vi "Connect LCR Relay.vi"(0 "reference in":refnum<class "NI-DAQmx.lvclass">, 2 "Relay Mode":enum16{"UV", "UW", "VW"}(ring), 5 "error in (no error)":errorcluster) -> (14 "reference out":refnum<class "NI-DAQmx.lvclass">, 19 "error out":errorcluster)   [LabVIEW 2018, in "NI-DAQmx.lvclass"]
uses:
  NI-DAQmx.lvclass
  <vilib>/DAQmx/write.llb/DAQmx Write (Digital 1D Bool NChan 1Samp 1Line).vi
  <vilib>/DAQmx/miscellaneous.llb/DAQmx Fill In Error Info.vi
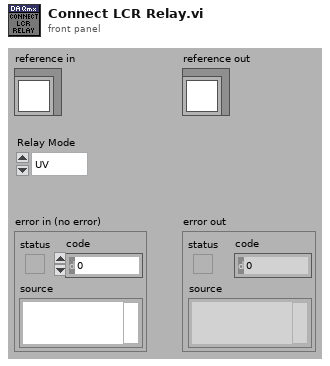
[diagram p1: front panel]
types:
  T1 = typedef "NI-DAQmx.lvclass/ObjectAttributes.ctl" = cluster{"AI Task":refnum<k21>, "DO Task":refnum<k21>, "AO Task":refnum<k21>, "Latest Values":dbl[], "Signal List":T2[], "PWM Duty Cycle (%)":dbl, "PWM Amplitude (V)":dbl, "PWM Frequency (Hz)":dbl, "DO States":bool[]}
  T2 = typedef "IO Signal List.ctl" = enum16{"Timestamp", "PSU_FB_U_VDC", "PSU_FB_I_AMP", "PSU_FB_W_WATT", "PSU_CMD_U_VDC", "PSU_CMD_I_AMP", "PSU_CMD_OUTPUT", "U_U_VDC", "V_U_VDC", "W_U_VDC", "U_I_AMP", "V_I_AMP", "W_I_AMP", "LCR_PRIMARY", "LCR_SECONDARY", "UV_R_mOhm", "UW_R_mOhm", "VW_R_mOhm", "UV_L_µH", "UW_L_µH", "VW_L_µH", "DIFF_UV_UW_L_µH", "DIFF_UV_VW_L_µH", "DIFF_UW_VW_L_µH", "DIFF_UV_UW_R_mOhm", "DIFF_UV_VW_R_mOhm", "DIFF_UW_VW_R_mOhm", "DIFF_UV_U_VDC", "DIFF_UW_U_VDC", "DIFF_VW_U_VDC", "PWM_CMD_DC_%", "PWM_CMD_VDC", "PWM_CMD_Hz", "PWM_FB_DC_%", "PWM_FB_VDC", "PWM_FB_Hz", "DO_RELAY_U_LCR_A", "DO_RELAY_V_LCR_A", "DO_RELAY_V_LCR_B", "DO_RELAY_W_LCR_B"}
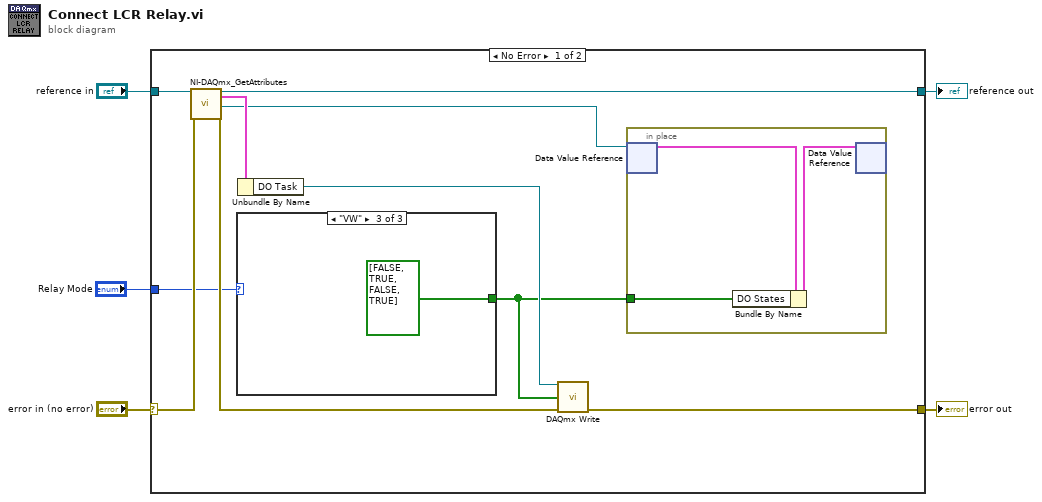
[diagram p0: block diagram]
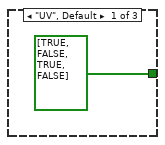
[diagram p2: hidden frame]
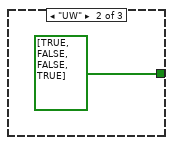
[diagram p3: hidden frame]
diagram:
  n1 = case shown="No Error" "error in (no error)" {
    selector: "error in (no error)" -> [w15 w23]
    tunnel: [w10 w23] -> w4
    tunnel: [w12 w22] -> w2
    tunnel: "reference in" -> [w13 w22]
    tunnel: "Relay Mode" -> [w8 _]
    frame No Error {
      n2 = call "NI-DAQmx_GetAttributes.vi"("reference in"=w13, "error in (no error)"=w15) -> ("reference out"=w12:refnum<class "NI-DAQmx.lvclass">, "Data"=w14:T1, "DataRef"=w7:refnum<data-value>, "error out"=w11:errorcluster)  [unwired: 14 in]
      n3 = case shown="\"VW\"" w8 {
        tunnel: [bool[] [TRUE, FALSE, TRUE, FALSE] ("data") bool[] [TRUE, FALSE, FALSE, TRUE] ("data") bool[] [FALSE, TRUE, FALSE, TRUE] ("data")] -> w6
        frame "UV", Default {
        }
        frame "UW" {
        }
        frame "VW" {
        }
      }
      n4 = Unbundle By Name(w14) -> ("DO Task"=w9:refnum<k21>)
      n5 = call-poly <vilib>:"DAQmx Write.vi"("task/channels in"=w9, "data"=w6, "error in"=w11) -> ("error out"=w10:errorcluster)  [unwired: 10 in, 2 out]
      n6 = in-place {
        in-place-border: w6 -> [w17]
        n7 = in-place-dvr #1(w7) -> (w18:T1)  [unwired: 1 out]
        n8 = Bundle By Name(cluster=w18, "DO States"=w17) -> (w16:T1)
        n9 = in-place-dvr #1(w16) -> ()  [unwired: 2 out]
      }
    }
    frame Error {
    }
  }
  "error out" <- w4
  "reference out" <- w2
